vi "ModifyAcc.vi"(8 "error in (no error)":errorcluster, 11 "UserManagement in":refnum<class "UserManagement.lvclass">) -> (0 "error out":errorcluster, 3 "UserManagement out":refnum<class "UserManagement.lvclass">)   [LabVIEW 2019, in "UserManagement.lvlib" / "UserManagement.lvclass"]
uses:
  UserManagement.lvclass
  UserManagement.lvclass/UserManagement.ctl
panel:
  in  "Cancel":bool
  in  "OK":bool
  in  "RepeatPassWord":string
  in  "PassWord":string
  out "UesrName":string
  in  "Privileges":enum16{"Engineer", "Technical", "Operator"}(ring)
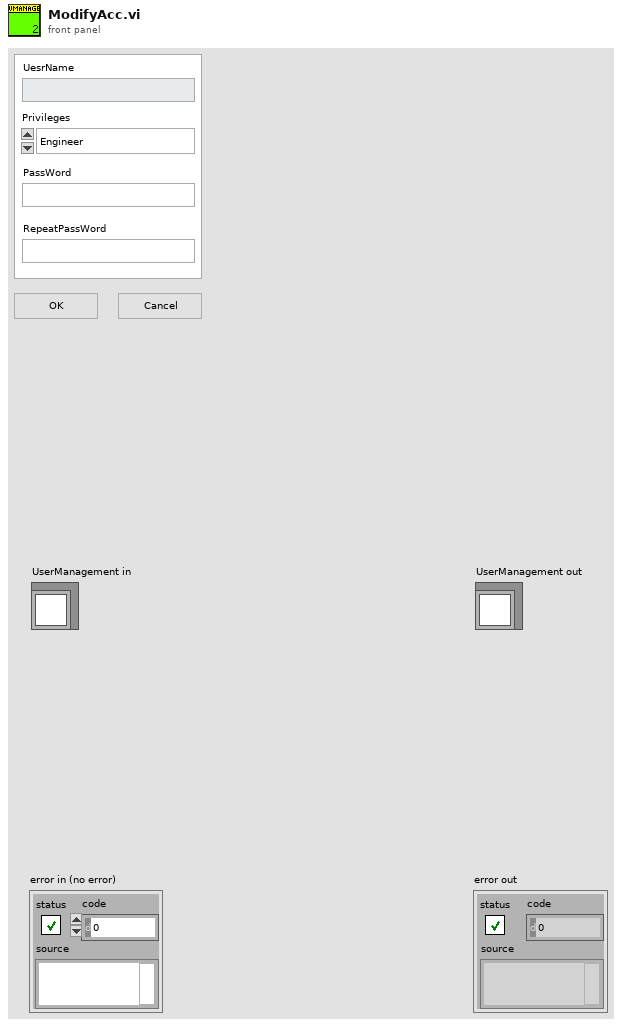
[diagram p1: front panel]
types:
  T1 = enum32{"Invalid", "Standard", "Closed", "Hidden", "Minimized", "Maximized"}
  T2 = enum32{"invalid app kind", "Development System", "Run Time System", "Student Edition", "Embedded LabVIEW", "Evaluation", "Custom"}
  T3 = cluster{"Core":cluster{"Current VI Reference":refnum<vi>, "Close Panel on Exit?":bool}, "Privileges":refnum<vi>, "Acc_Info_Str":string[][], "UserName":string, "Index":i32}
  T4 = cluster{"Current VI Reference":refnum<vi>, "Close Panel on Exit?":bool}
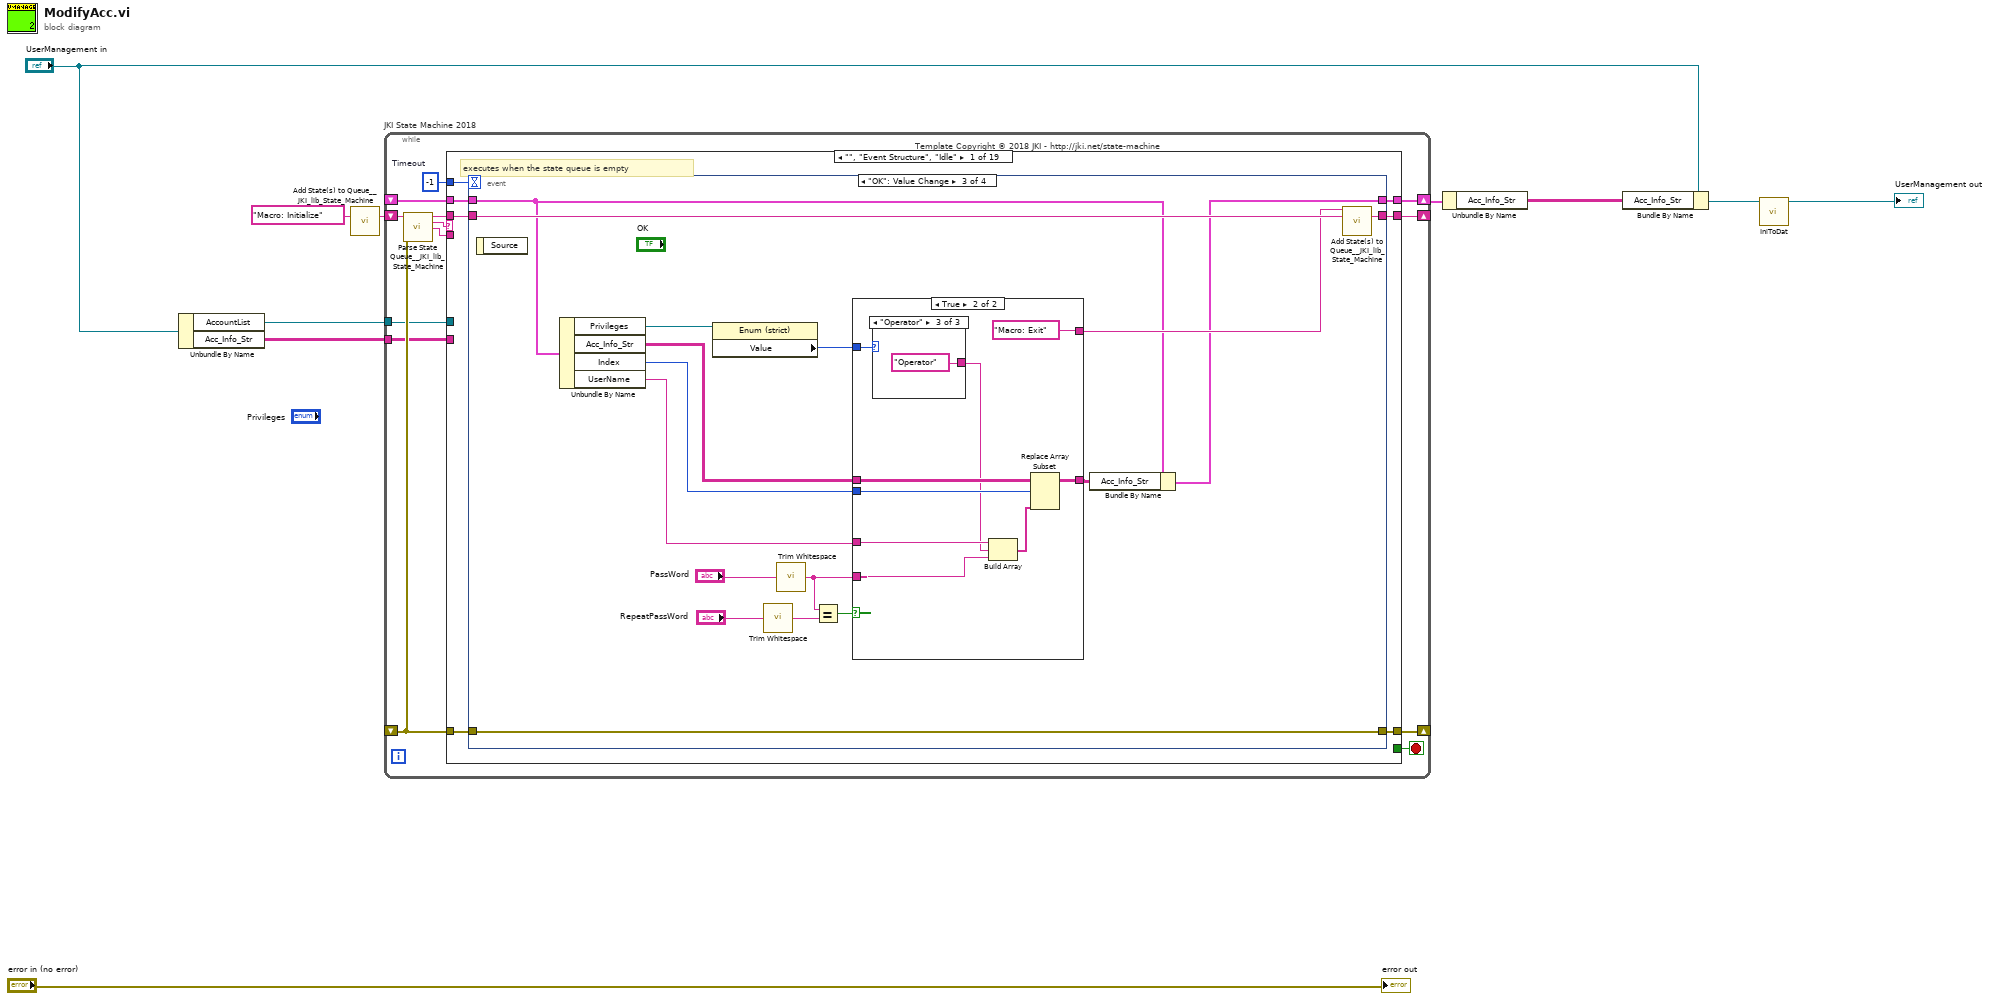
[diagram p0: block diagram]
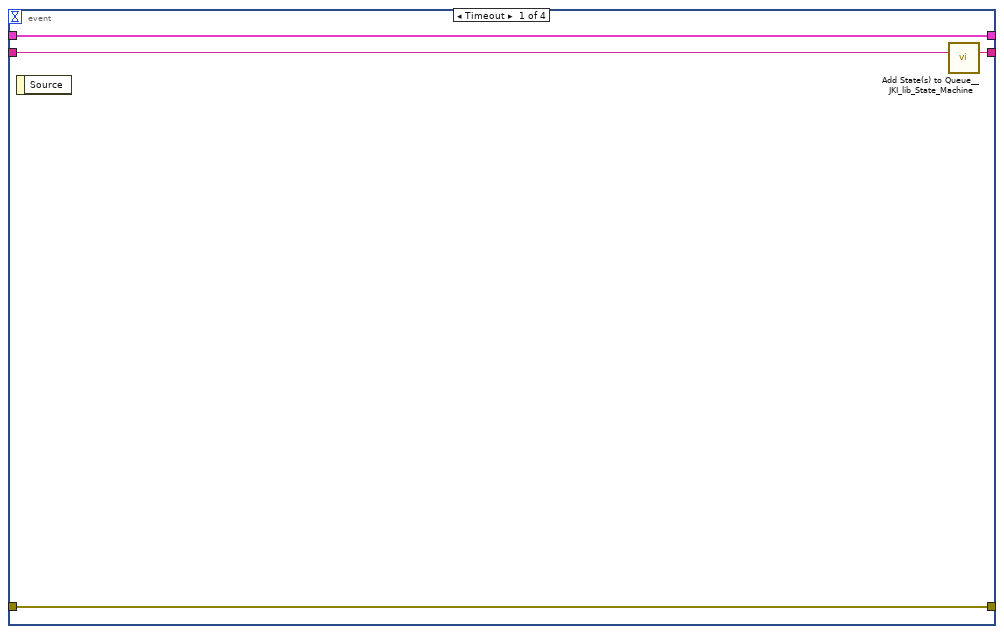
[diagram p2: hidden frame]
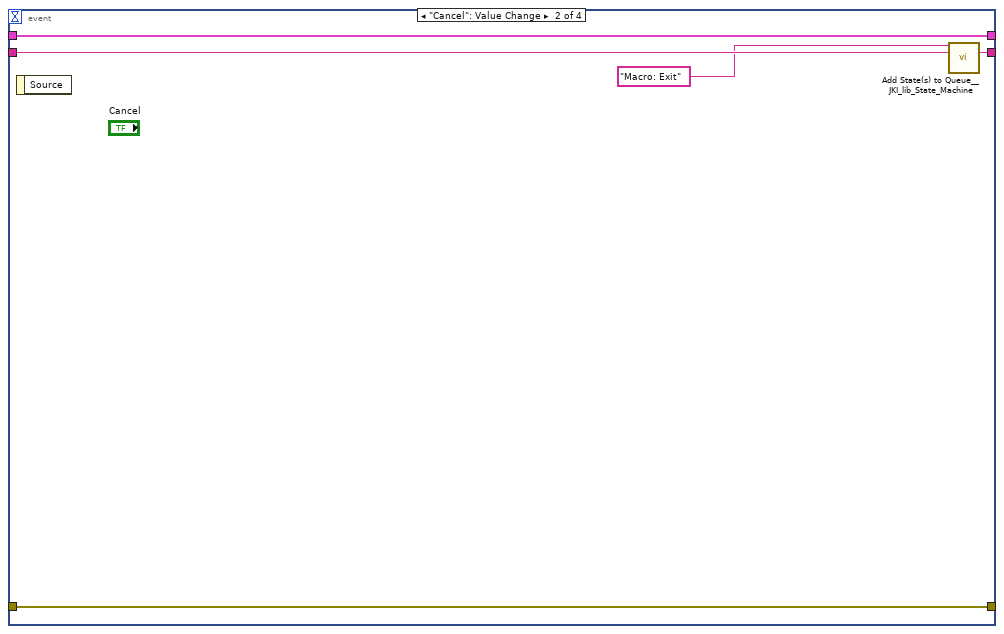
[diagram p3: hidden frame]
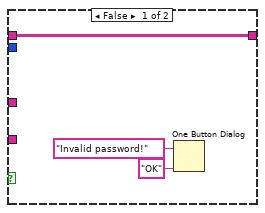
[diagram p4: hidden frame]
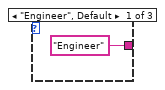
[diagram p5: hidden frame]
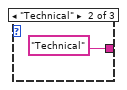
[diagram p6: hidden frame]
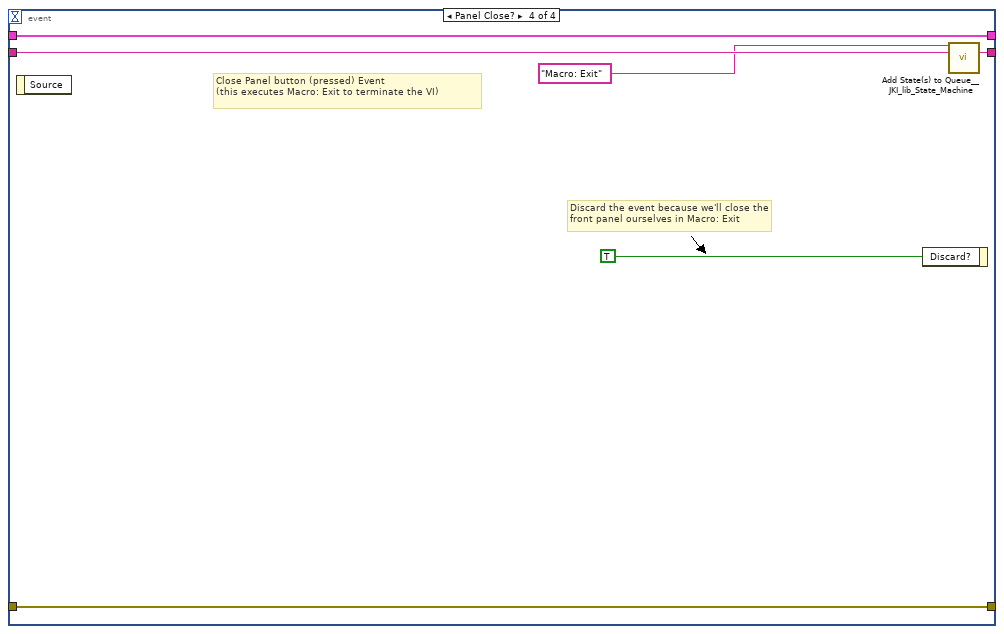
[diagram p7: hidden frame]
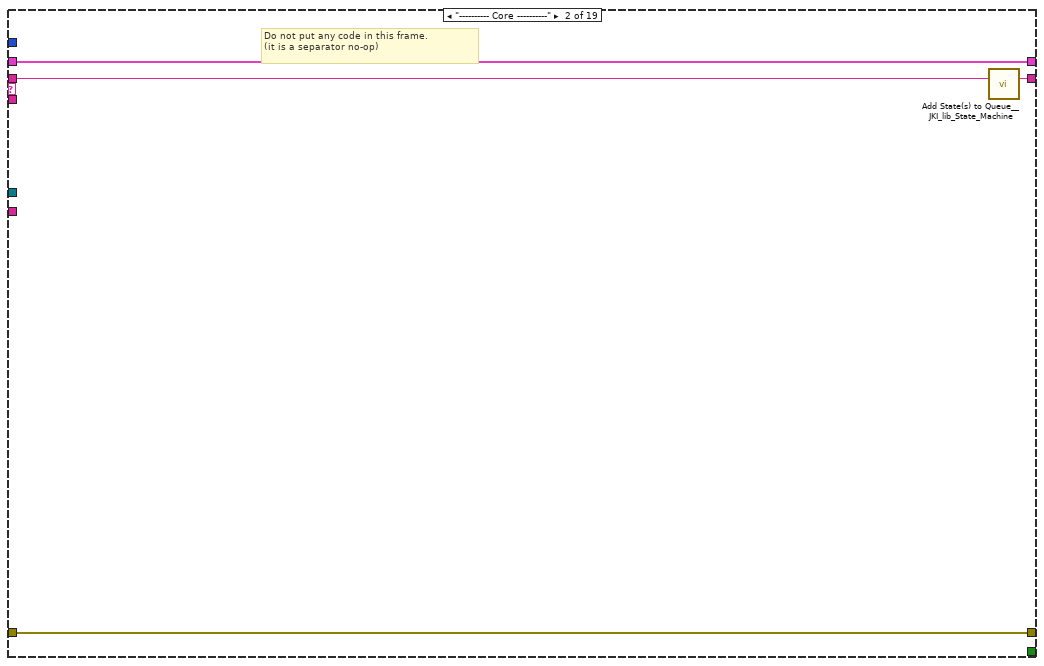
[diagram p8: hidden frame]
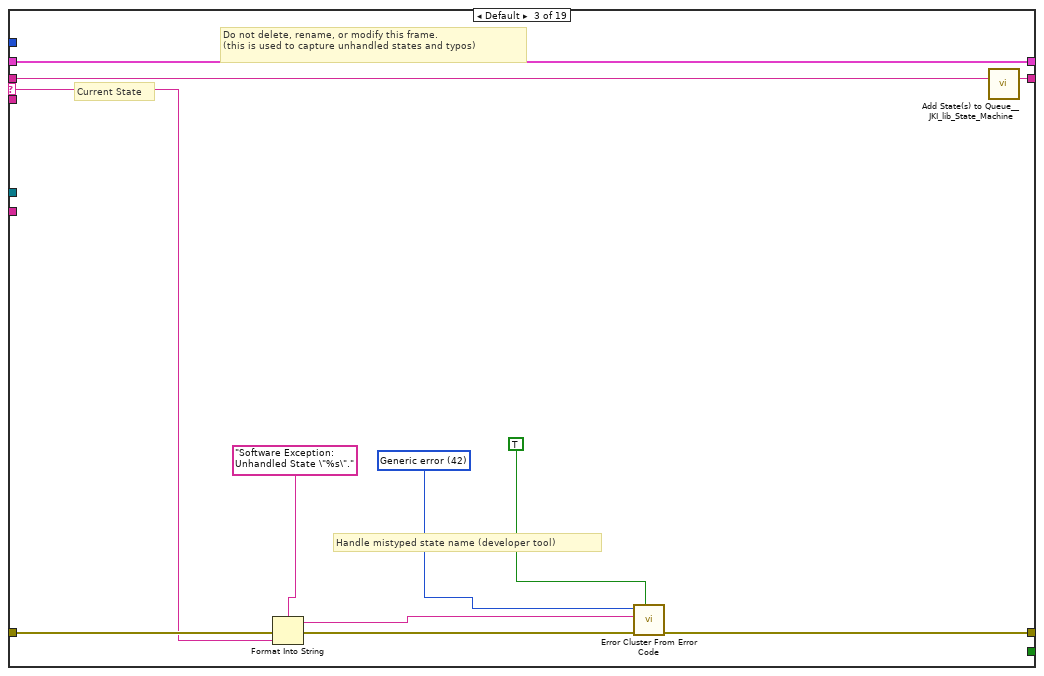
[diagram p9: hidden frame]
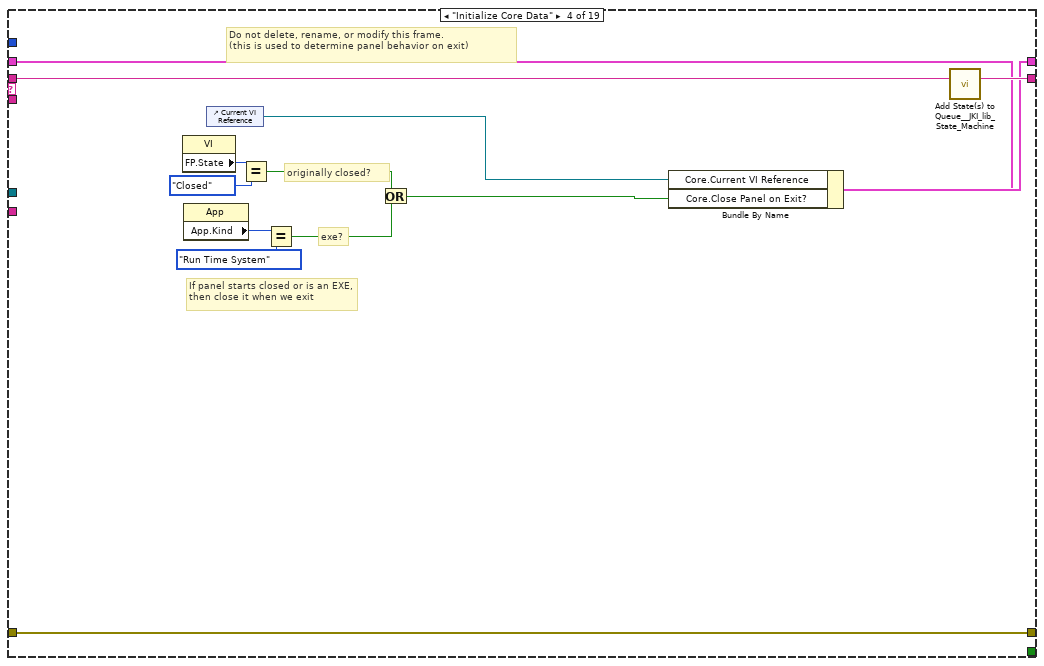
[diagram p10: hidden frame]
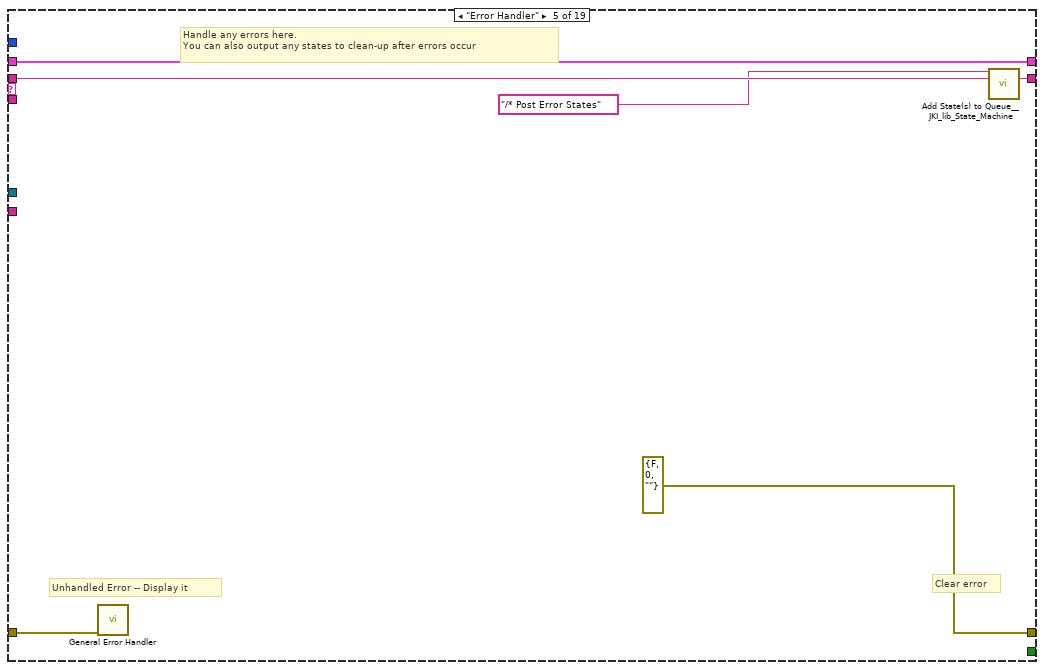
[diagram p11: hidden frame]
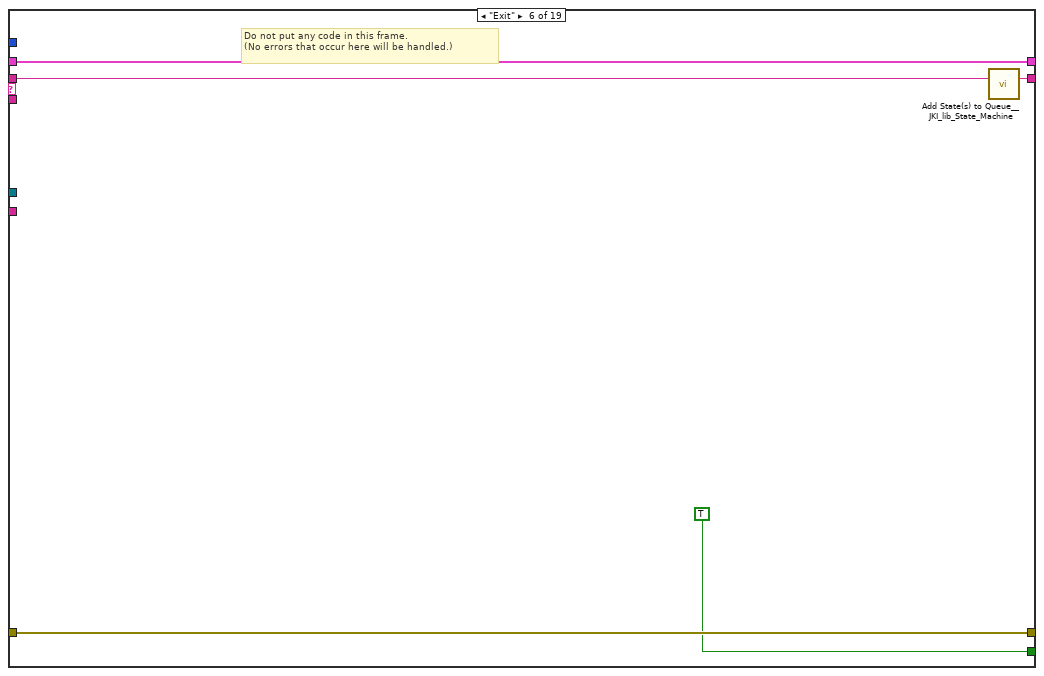
[diagram p12: hidden frame]
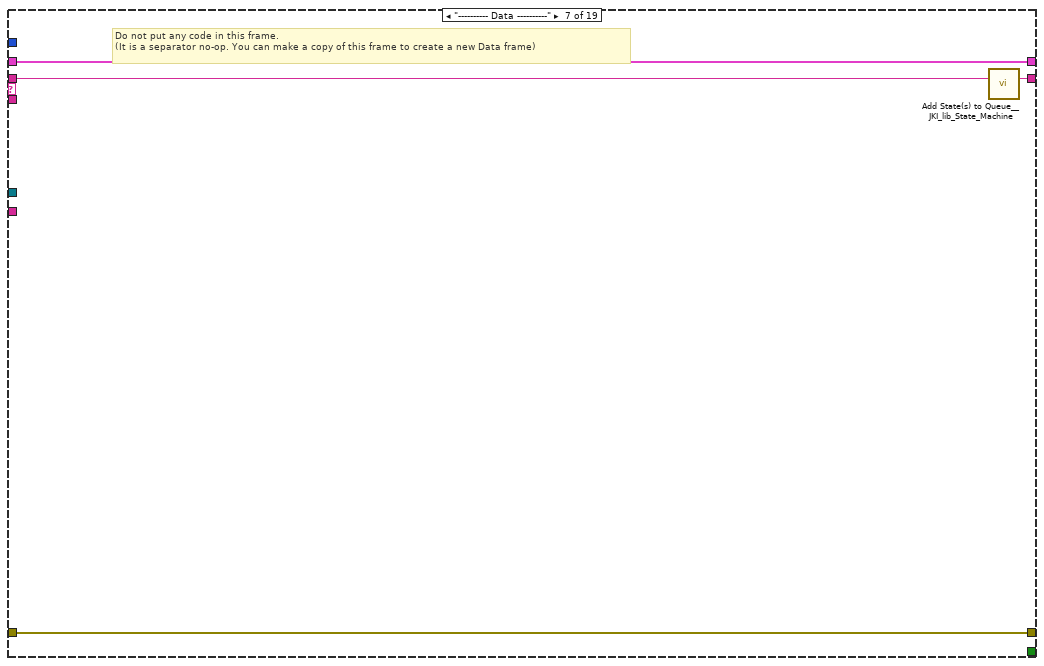
[diagram p13: hidden frame]
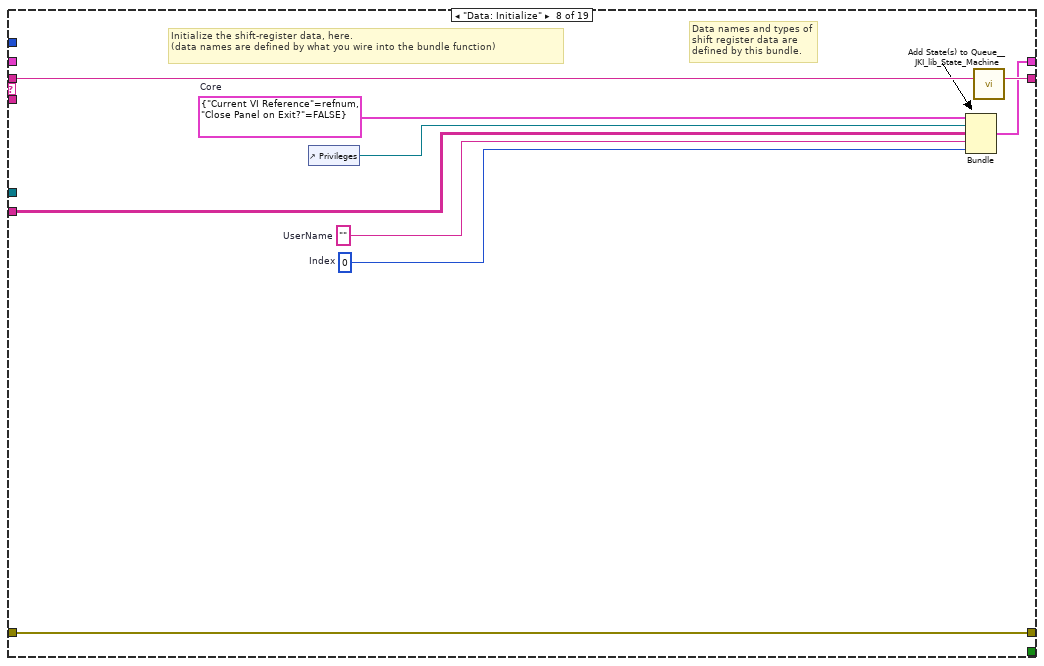
[diagram p14: hidden frame]
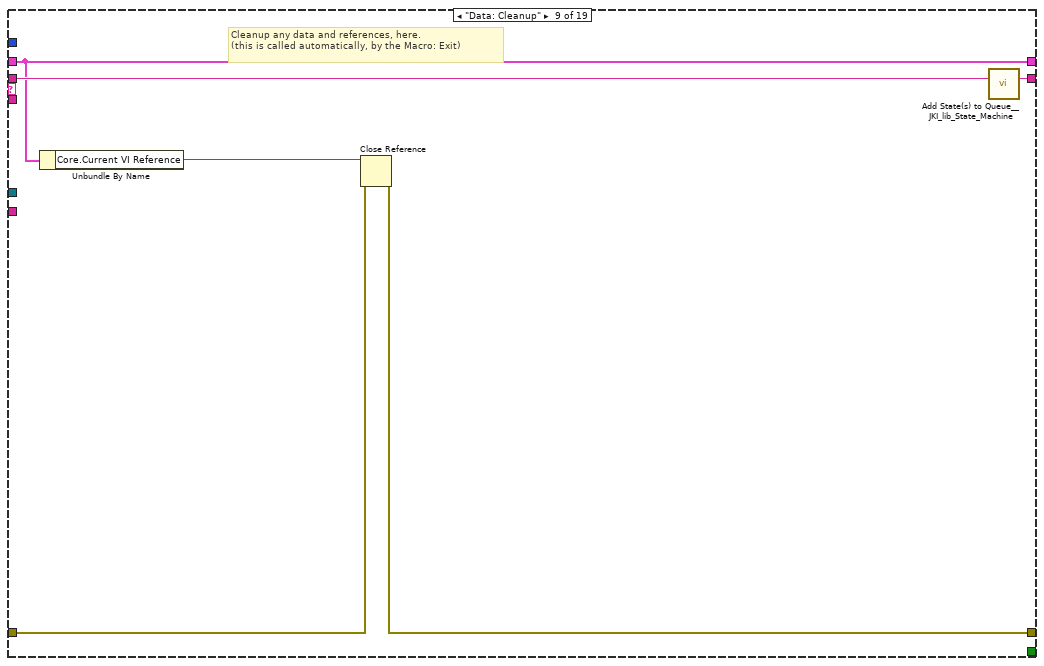
[diagram p15: hidden frame]
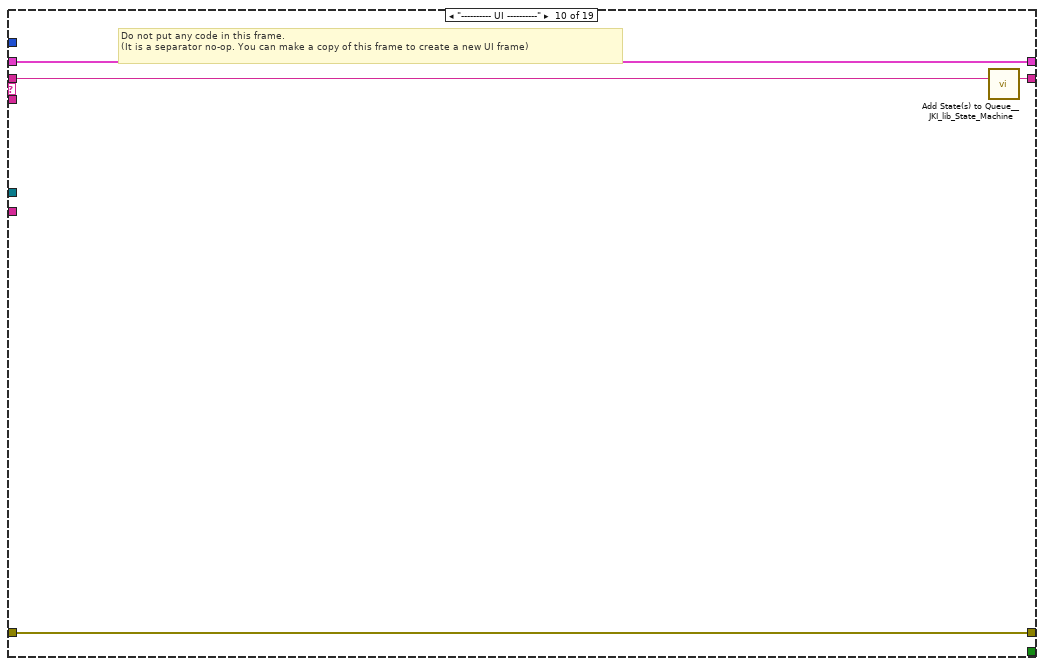
[diagram p16: hidden frame]
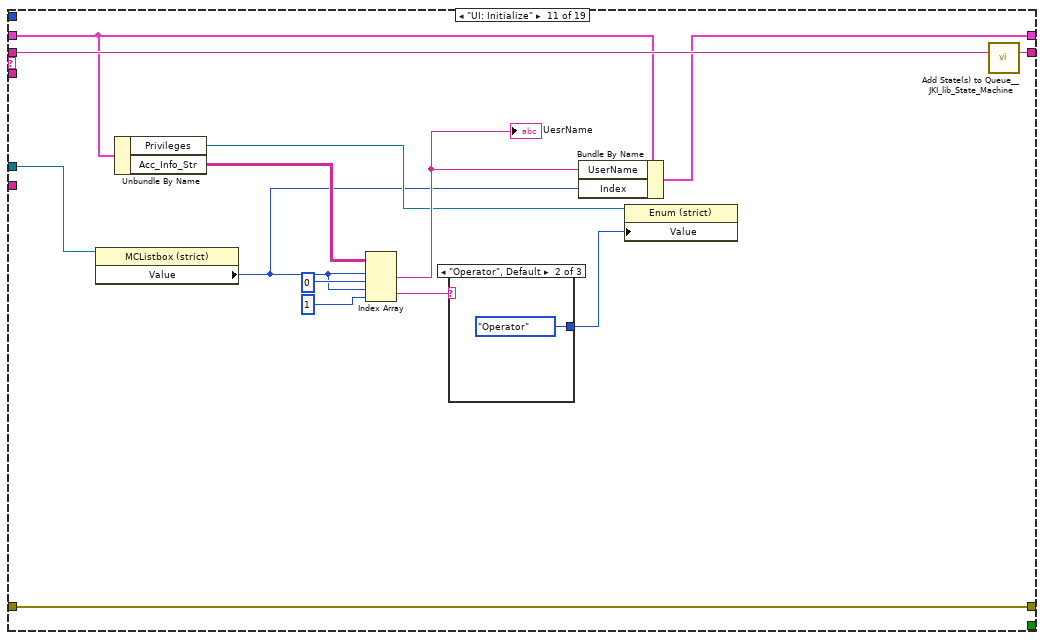
[diagram p17: hidden frame]
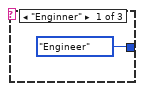
[diagram p18: hidden frame]
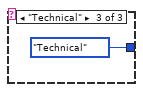
[diagram p19: hidden frame]
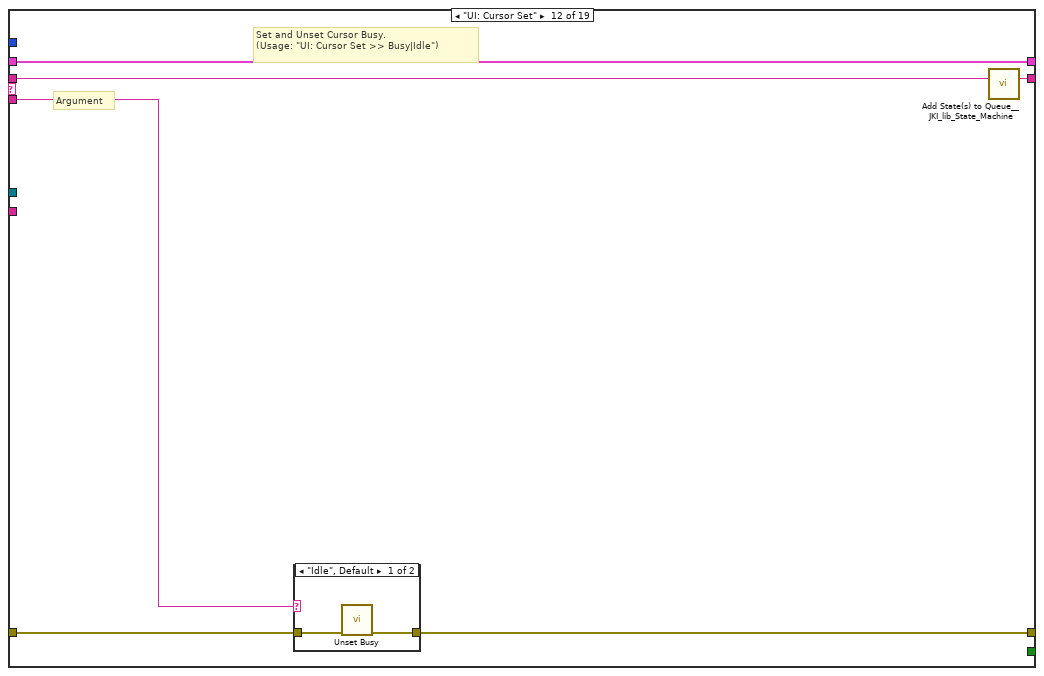
[diagram p20: hidden frame]
diagram:
  n1 = Unbundle By Name("UserManagement in") -> ("AccountList"=w7:refnum<vi>, "Acc_Info_Str"=w6:string[][])
  n2 = call <vilib>:"Add State(s) to Queue__JKI_lib_State_Machine.vi"("State(s) in (\"\")"="Macro: Initialize") -> ("States Out"=w9:string)  [unwired: 14 in]
  n3 = while "JKI State Machine 2018" {
    shift-right: [w16] -> w5
    shift-left: _ -> [w15]
    shift-right: [w19] -> _
    shift-left: _ -> [w13]
    shift-right: [w18] -> _
    shift-left: w9 -> [w20]
    tunnel: w7 -> [w12]
    tunnel: w6 -> [w11]
    stop <- w17 stop-if-true
    w14 = -1  # Timeout
    # "Template Copyright © 2018 JKI - http://jki.net/state-machine"
    n4 = call <vilib>:"Parse State Queue__JKI_lib_State_Machine.vi"("State Queue"=w20, "Error In (no error)"=w13) -> ("Remaining States"=w22:string, "Current State"=w23:string, "Arguments"=w21:string)  [unwired: 11 in]
    n5 = case shown="\"\", \"Event Structure\", \"Idle\"" w23 {
      selector: w23 -> [_ _ w82 _ _ _ _ _ _ _ _ _ _ _ _ _ _ _ _]
      tunnel: w22 -> [w30 w81 w86 w105 w111 w116 w120 w129 w135 w139 w153 w162 w173 w242 w247 w257 w261 w265 w269]
      tunnel: w21 -> [_ _ _ _ _ _ _ _ _ _ _ w157 w167 _ _ _ _ _ _]
      tunnel: w15 -> [w28 w78 w84 w98 w108 w114 w117 _ w130 w136 w144 w160 w169 w239 w244 w254 w258 w262 w266]
      tunnel: [w27 w79 w88 w102 errorcluster {"status"=FALSE, "code"=0, "source"=""} ("error out") w113 w118 w126 w131 w137 w151 w158 w170 w240 w245 w255 w259 w263 w267] -> w19
      tunnel: w13 -> [w26 w79 w87 w102 w107 w113 w118 w126 w132 w137 w151 w159 w171 w240 w245 w255 w259 w263 w267]
      tunnel: [w29 w80 w85 w104 w110 w115 w119 w128 w134 w138 w152 w161 w172 w241 w246 w256 w260 w264 w268] -> w18
      tunnel: [_ _ _ _ _ TRUE _ _ _ _ _ _ _ _ _ _ _ _ _] -> w17
      tunnel: [w25 w78 w84 w103 w108 w114 w117 w127 w130 w136 w141 w160 w169 w239 w244 w254 w258 w262 w266] -> w16
      tunnel: w14 -> [w24 _ _ _ _ _ _ _ _ _ _ _ _ _ _ _ _ _ _]
      tunnel: w12 -> [_ _ _ _ _ _ _ _ _ _ w142 _ _ _ _ _ _ _ _]
      tunnel: w11 -> [_ _ _ _ _ _ _ w123 _ _ _ _ _ _ _ _ _ _ _]
      frame "", "Event Structure", "Idle" {
        # "executes when the state queue is empty"
        n6 = event shown="[2] \"OK\": Value Change" {
          selector: _ -> [_ _ _ _]
          dyn-events: _ -> [_ _ _ _]
          timeout: w24 -> [_ _ _ _]
          tunnel: w30 -> [w34 w39 w56 w77]
          tunnel: [w33 w38 w55 w76] -> w29
          tunnel: w28 -> [w31 w36 w41 w74]
          tunnel: [w32 w37 w54 w75] -> w27
          tunnel: w26 -> [w32 w37 w54 w75]
          tunnel: [w31 w36 w40 w74] -> w25
          event Timeout {
            n7 = event-data() -> ()  [unwired: 1 in, 1 out]
            n8 = call <vilib>:"Add State(s) to Queue__JKI_lib_State_Machine.vi"("State(s) in (\"\")"=w34) -> ("States Out"=w33:string)  [unwired: 14 in]
          }
          event "Cancel": Value Change {
            n9 = event-data() -> ()  [unwired: 1 in, 1 out]
            n10 = call <vilib>:"Add State(s) to Queue__JKI_lib_State_Machine.vi"("State(s) in Front (\"\")"="Macro: Exit", "State(s) in (\"\")"=w39) -> ("States Out"=w38:string)  [unwired: 13 in]
          }
          event "OK": Value Change {
            n11 = event-data() -> ()  [unwired: 1 in, 1 out]
            n12 = Unbundle By Name(w41) -> ("Privileges"=w46:refnum<vi>, "Acc_Info_Str"=w45:string[][], "Index"=w44:i32, "UserName"=w43:string)
            n13 = property class="Enum (strict)"(reference=w46) -> ("Value"=w50:enum16{"Engineer", "Technical", "Operator"})  [unwired: 1 in, 2 out]
            n14 = call <vilib>:"Trim Whitespace.vi"("string"="RepeatPassWord") -> ("trimmed string"=w53:string)  [unwired: 1 in]
            n15 = call <vilib>:"Trim Whitespace.vi"("string"="PassWord") -> ("trimmed string"=w51:string)  [unwired: 1 in]
            n16 = Equal?(x=w51, y=w53) -> (x = y?=w52:bool)
            n17 = case shown="True" w52 {
              tunnel: w45 -> [w59 w68]
              tunnel: w44 -> [_ w67]
              tunnel: w51 -> [_ w62]
              tunnel: w43 -> [_ w64]
              tunnel: w50 -> [_ w66]
              tunnel: [w59 w65] -> w49
              tunnel: [_ "Macro: Exit"] -> w42
              frame False {
                n18 = One Button Dialog(message="Invalid password!" ("消息"), button name ("OK")="OK" ("按钮名称（“确定”）")) -> ()  [unwired: 1 out]
              }
              frame True {
                n19 = case shown="\"Operator\"" w66 {
                  tunnel: ["Engineer" "Technical" "Operator"] -> w63
                  frame "Engineer", Default {
                  }
                  frame "Technical" {
                  }
                  frame "Operator" {
                  }
                }
                n20 = Build Array(w64, w63, w62) -> (w61:string[])
                n21 = Replace Array Subset(array=w68, new element=w61, index (row)=w67) -> (w65:string[][])  [unwired: 1 in]
              }
            }
            n22 = Bundle By Name(cluster=w41, "Acc_Info_Str"=w49) -> (w40:T3)
            n23 = call <vilib>:"Add State(s) to Queue__JKI_lib_State_Machine.vi"("State(s) in Front (\"\")"=w42, "State(s) in (\"\")"=w56) -> ("States Out"=w55:string)  [unwired: 13 in]
          }
          event Panel Close? {
            # "Discard the event because we'll close the front panel ourselves in Macro: Exit"
            # "Close Panel button (pressed) Event\n(this executes Macro: Exit to terminate the VI)"
            n24 = event-data() -> ()  [unwired: 1 in, 1 out]
            n25 = event-data("Discard?"=TRUE) -> ()  [unwired: 1 in, 1 out]
            n26 = call <vilib>:"Add State(s) to Queue__JKI_lib_State_Machine.vi"("State(s) in Front (\"\")"="Macro: Exit", "State(s) in (\"\")"=w77) -> ("States Out"=w76:string)  [unwired: 13 in]
          }
        }
      }
      frame "---------- Core ----------" {
        # "Do not put any code in this frame.\n(it is a separator no-op)"
        n27 = call <vilib>:"Add State(s) to Queue__JKI_lib_State_Machine.vi"("State(s) in (\"\")"=w81) -> ("States Out"=w80:string)  [unwired: 14 in]
      }
      frame Default {
        w91 = 42 items=["No error", "Argument error", "Memory is full", "Out of zone", "End of file", "File already open", "Generic file I/O error", "File not found", "File permission error", "Disk is full", "Duplicate path", "Too many files open", "System feature not enabled", "Resource file not found", "Cannot add resource", "Resource not found", "Image not found", "Image memory error", "Pen does not exist", "Config type invalid", "Config token not found", "Config parse error", "Config memory error", "Bad external code format", "Bad external code offset", "External code not present", "Null window", "Destroy window error", "Null menu", "Print aborted", "Bad print record", "Print driver error", "Windows error during printing", "Memory error during printing", "Print dialog error", "Generic print error", "Invalid device refnum", "Device not found", "Device parameter error", "Device unit error", "Cannot open device", "Device call aborted", "Generic error", "Cancelled by user", "Object ID too low", "Object ID too high", "Object not in heap", "Unknown heap", "Unknown object (invalid DefProc)", "Unknown object (DefProc not in table)", "Message out of range", "Invalid (null) method", "Unknown message", "Manager call not supported", "Bad address", "Network operation in progress", "Network operation timed out", "Connection is busy", "Network attribute not supported", "Network error", "Address in use", "System out of memory", "Connection aborted", "Connection refused", "Not connected", "Already connected", "Connection closed", "Initialization error (interapplication manager)", "Bad occurrence", "Wait on unbound occurrence handler", "Occurrence queue overflow", "Datalog type conflict", "Unused", "Unrecognized type (interapplication manager)", "Memory corrupt", "Failed to make temporary DLL", "Old CIN version", "Drag socket not found", "Failed to load drop-object", "Failed to register OLE object", "Failed to release OLE object", "Format specifier type mismatch", "Unknown format specifier", "Too few format specifiers", "Too many format specifiers", "Scan failed", "Newer CIN version", "Error converting to variant", "Runtime menu error", "Password tampered", "Variant attribute not found", "Incompatible variant data type", "Event data is not available", "Event Store is not present", "Occurrence is not found", "Event Queue is not created", "Event info is not available", "Refnum passed is NULL", "Error retrieving Class GUID", "Error retrieving CoClass GUID", "Error retrieving TypeLib GUID.", "Bad built application magic bytes.", "Specific driver is different from the specific driver associated with the Logical Name.", "There is no session opened to the class driver.", "Max Error", "MAX - Error with config objects", "MAX - Error loading configuration", "MAX - Group not supported"]
        # "Current State"
        # "Do not delete, rename, or modify this frame.\n(this is used to capture unhandled states and typos)"
        # "Handle mistyped state name (developer tool)"
        n28 = Format Into String(format string="Software Exception: Unhandled State \"%s\"." ("message"), error in=w87, w82) -> (resulting string=w90:string, error out=w89:errorcluster)  [unwired: 1 in]
        n29 = call <vilib>:"Error Cluster From Error Code.vi"("show call chain? (False)"=TRUE, "error in (no error)"=w89, "error message (\"\")"=w90, "error code (0)"=w91) -> ("error out"=w88:errorcluster)  [unwired: 5 in]
        n30 = call <vilib>:"Add State(s) to Queue__JKI_lib_State_Machine.vi"("State(s) in (\"\")"=w86) -> ("States Out"=w85:string)  [unwired: 14 in]
      }
      frame "Initialize Core Data" {
        # "Do not delete, rename, or modify this frame.\n(this is used to determine panel behavior on exit)"
        # "originally closed?"
        # "exe?"
        # "If panel starts closed or is an EXE, then close it when we exit"
        n31 = property class="VI"() -> ("FP.State"=w95:T1)  [unwired: 2 in, 2 out]
        n32 = property class="App"() -> ("App.Kind"=w101:T2)  [unwired: 2 in, 2 out]
        n33 = control-ref of="Current VI Reference"() -> (w96:refnum<vi>)
        n34 = Equal?(x=w95, y=T1."Closed" ("Front Panel Window:State")) -> (x = y?=w93:bool)
        n35 = Equal?(x=w101, y=T2."Run Time System" ("Application:Kind")) -> (x = y?=w99:bool)
        n36 = Or(x=w93, y=w99) -> (x .or. y?=w97:bool)
        n37 = Bundle By Name(cluster=w98, "Core.Current VI Reference"=w96, "Core.Close Panel on Exit?"=w97) -> (w103:T3)
        n38 = call <vilib>:"Add State(s) to Queue__JKI_lib_State_Machine.vi"("State(s) in (\"\")"=w105) -> ("States Out"=w104:string)  [unwired: 14 in]
      }
      frame "Error Handler" {
        # "Unhandled Error -- Display it"
        # "Handle any errors here.\nYou can also output any states to clean-up after errors occur"
        # "Clear error"
        n39 = call <vilib>:"General Error Handler.vi"("error in (no error)"=w107) -> ()  [unwired: 10 in, 5 out]
        n40 = call <vilib>:"Add State(s) to Queue__JKI_lib_State_Machine.vi"("State(s) in Front (\"\")"="/* Post Error States", "State(s) in (\"\")"=w111) -> ("States Out"=w110:string)  [unwired: 13 in]
      }
      frame "Exit" {
        # "Do not put any code in this frame.\n(No errors that occur here will be handled.)"
        n41 = call <vilib>:"Add State(s) to Queue__JKI_lib_State_Machine.vi"("State(s) in (\"\")"=w116) -> ("States Out"=w115:string)  [unwired: 14 in]
      }
      frame "---------- Data ----------" {
        # "Do not put any code in this frame.\n(It is a separator no-op. You can make a copy of this frame to create a new Data frame)"
        n42 = call <vilib>:"Add State(s) to Queue__JKI_lib_State_Machine.vi"("State(s) in (\"\")"=w120) -> ("States Out"=w119:string)  [unwired: 14 in]
      }
      frame "Data: Initialize" {
        w121 = 0  # Index
        w122 = ""  # UserName
        w125 = T4 {"Current VI Reference"=refnum, "Close Panel on Exit?"=FALSE}  # Core
        # "Data names and types of shift register data are defined by this bundle."
        # "Initialize the shift-register data, here.\n(data names are defined by what you wire into the bundle function)"
        n43 = control-ref of="Privileges"() -> (w124:refnum<vi>)
        n44 = Bundle("Core"=w125, "Privileges"=w124, "Acc_Info_Str"=w123, "UserName"=w122, "Index"=w121) -> (w127:T3)  [unwired: 1 in]
        n45 = call <vilib>:"Add State(s) to Queue__JKI_lib_State_Machine.vi"("State(s) in (\"\")"=w129) -> ("States Out"=w128:string)  [unwired: 14 in]
      }
      frame "Data: Cleanup" {
        # "Cleanup any data and references, here.\n(this is called automatically, by the Macro: Exit)"
        n46 = Unbundle By Name(w130) -> ("Core.Current VI Reference"=w133:refnum<vi>)
        n47 = Close Reference(reference=w133, error in (no error)=w132) -> (error out=w131:errorcluster)
        n48 = call <vilib>:"Add State(s) to Queue__JKI_lib_State_Machine.vi"("State(s) in (\"\")"=w135) -> ("States Out"=w134:string)  [unwired: 14 in]
      }
      frame "---------- UI ----------" {
        # "Do not put any code in this frame.\n(It is a separator no-op. You can make a copy of this frame to create a new UI frame)"
        n49 = call <vilib>:"Add State(s) to Queue__JKI_lib_State_Machine.vi"("State(s) in (\"\")"=w139) -> ("States Out"=w138:string)  [unwired: 14 in]
      }
      frame "UI: Initialize" {
        n50 = property class="MCListbox (strict)"(reference=w142) -> ("Value"=w140:i32)  [unwired: 1 in, 2 out]
        n51 = Unbundle By Name(w144) -> ("Privileges"=w145:refnum<vi>, "Acc_Info_Str"=w143:string[][])
        n52 = Index Array(array=w143, index (row) #1=w140, index (col) #1=0 ("禁用的索引 (列)"), index (row) #2=w140, index (col) #2=1 ("禁用的索引 (列)")) -> (element #1=w146:string, element #2=w148:string)
        "UesrName" <- w146
        n53 = case shown="\"Operator\", Default" w148 {
          tunnel: [enum16{"Engineer", "Technical", "Operator"}."Engineer" ("Value") enum16{"Engineer", "Technical", "Operator"}."Operator" ("Value") enum16{"Engineer", "Technical", "Operator"}."Technical" ("Value")] -> w147
          frame "Enginner" {
          }
          frame "Operator", Default {
          }
          frame "Technical" {
          }
        }
        n54 = Bundle By Name(cluster=w144, "UserName"=w146, "Index"=w140) -> (w141:T3)
        n55 = property class="Enum (strict)"(reference=w145, "Value"=w147) -> ()  [unwired: 1 in, 2 out]
        n56 = call <vilib>:"Add State(s) to Queue__JKI_lib_State_Machine.vi"("State(s) in (\"\")"=w153) -> ("States Out"=w152:string)  [unwired: 14 in]
      }
      frame "UI: Cursor Set" {
        # "Argument"
        # "Set and Unset Cursor Busy.\n(Usage: \"UI: Cursor Set >> Busy|Idle\")"
        n57 = case shown="\"Idle\", Default" w157 {
          tunnel: w159 -> [w164 w166]
          tunnel: [w163 w165] -> w158
          frame "Idle", Default {
            n58 = call <vilib>:"Unset Busy.vi"("error in (no error)"=w164) -> ("error out"=w163:errorcluster)  [unwired: 10 in]
          }
          frame "Busy" {
            n59 = call <vilib>:"Set Busy.vi"("error in (no error)"=w166) -> ("error out"=w165:errorcluster)  [unwired: 9 in, 1 out]
          }
        }
        n60 = call <vilib>:"Add State(s) to Queue__JKI_lib_State_Machine.vi"("State(s) in (\"\")"=w162) -> ("States Out"=w161:string)  [unwired: 14 in]
      }
      frame "UI: Front Panel State" {
        # "Argument"
        # "Set Front Panel Open or Closed\n(Usage: \"UI: Front Panel State >> Open|Close\")"
        n61 = Unbundle By Name(w169) -> ("Core.Current VI Reference"=w168:refnum<vi>)
        n62 = case shown="\"Minimize\", \"Minimized\"" w167 {
          tunnel: w171 -> [w179 w194 w205 w218 w231]
          tunnel: [w181 w195 w207 w220 w233] -> w170
          tunnel: w168 -> [w180 w192 w206 w219 w232]
          frame "Open", "Standard", Default {
            w174 = T1."Standard" ("State")
            n63 = property class="VI"(reference=w180, error in=w179) -> (reference out=w177:refnum<vi>, error out=w178:errorcluster, "FP.State"=w176:T1)
            n64 = Not Equal?(x=w176, y=w174) -> (x != y?=w175:bool)
            n65 = case shown="True" w175 {
              tunnel: [w185 w187] -> w181
              tunnel: w178 -> [w184 w187]
              tunnel: w177 -> [w183 _]
              tunnel: w174 -> [w182 _]
              frame True {
                n66 = invoke class="VI" method="FP.Open"(reference=w183, error in=w184, "Activate"=TRUE, "State"=w182) -> (error out=w185:errorcluster)  [unwired: 1 in, 4 out]
              }
              frame False {
              }
            }
          }
          frame "Close", "Closed" {
            n67 = property class="VI"(reference=w192, error in=w194) -> (reference out=w191:refnum<vi>, error out=w193:errorcluster, "FP.State"=w189:T1)
            n68 = Not Equal?(x=w189, y=T1."Closed" ("Front Panel Window:State")) -> (x != y?=w188:bool)
            n69 = case shown="True" w188 {
              tunnel: [w196 w199] -> w195
              tunnel: w193 -> [w196 w198]
              tunnel: w191 -> [_ w197]
              frame False {
              }
              frame True {
                n70 = invoke class="VI" method="FP.Close"(reference=w197, error in=w198) -> (error out=w199:errorcluster)  [unwired: 1 in, 2 out]
              }
            }
          }
          frame "Hidden", "Hide" {
            w200 = T1."Hidden" ("State")
            n71 = property class="VI"(reference=w206, error in=w205) -> (reference out=w203:refnum<vi>, error out=w204:errorcluster, "FP.State"=w202:T1)
            n72 = Not Equal?(x=w202, y=w200) -> (x != y?=w201:bool)
            n73 = case shown="True" w201 {
              tunnel: [w211 w212] -> w207
              tunnel: w204 -> [w210 w212]
              tunnel: w203 -> [w209 _]
              tunnel: w200 -> [w208 _]
              frame True {
                n74 = invoke class="VI" method="FP.Open"(reference=w209, error in=w210, "State"=w208) -> (error out=w211:errorcluster)  [unwired: 2 in, 4 out]
              }
              frame False {
              }
            }
          }
          frame "Minimize", "Minimized" {
            w213 = T1."Minimized" ("State")
            n75 = property class="VI"(reference=w219, error in=w218) -> (reference out=w216:refnum<vi>, error out=w217:errorcluster, "FP.State"=w215:T1)
            n76 = Not Equal?(x=w215, y=w213) -> (x != y?=w214:bool)
            n77 = case shown="True" w214 {
              tunnel: [w224 w225] -> w220
              tunnel: w217 -> [w223 w225]
              tunnel: w216 -> [w222 _]
              tunnel: w213 -> [w221 _]
              frame True {
                n78 = invoke class="VI" method="FP.Open"(reference=w222, error in=w223, "State"=w221) -> (error out=w224:errorcluster)  [unwired: 2 in, 4 out]
              }
              frame False {
              }
            }
          }
          frame "Maximize", "Maximized" {
            w226 = T1."Maximized" ("State")
            n79 = property class="VI"(reference=w232, error in=w231) -> (reference out=w229:refnum<vi>, error out=w230:errorcluster, "FP.State"=w228:T1)
            n80 = Not Equal?(x=w228, y=w226) -> (x != y?=w227:bool)
            n81 = case shown="True" w227 {
              tunnel: [w237 w238] -> w233
              tunnel: w230 -> [w236 w238]
              tunnel: w229 -> [w235 _]
              tunnel: w226 -> [w234 _]
              frame True {
                n82 = invoke class="VI" method="FP.Open"(reference=w235, error in=w236, "State"=w234) -> (error out=w237:errorcluster)  [unwired: 2 in, 4 out]
              }
              frame False {
              }
            }
          }
        }
        n83 = call <vilib>:"Add State(s) to Queue__JKI_lib_State_Machine.vi"("State(s) in (\"\")"=w173) -> ("States Out"=w172:string)  [unwired: 14 in]
      }
      frame "---------- Macro ----------" {
        # "Do not put any code in this frame.\n(It is a separator no-op. You can make a copy of this frame to create a new Macro frame)"
        n84 = call <vilib>:"Add State(s) to Queue__JKI_lib_State_Machine.vi"("State(s) in (\"\")"=w242) -> ("States Out"=w241:string)  [unwired: 14 in]
      }
      frame "Macro: Initialize" {
        w243 = "Data: Initialize\nInitialize Core Data\nUI: Initialize\nUI: Front Panel State >> Open"  # Data: Initialize Initialize Core Data UI: Initialize UI: Front Panel State >> Open
        # "Initialization Macro\n(This is called once, when the VI starts)"
        n85 = call <vilib>:"Add State(s) to Queue__JKI_lib_State_Machine.vi"("State(s) in Front (\"\")"=w243, "State(s) in (\"\")"=w247) -> ("States Out"=w246:string)  [unwired: 13 in]
      }
      frame "Macro: Exit" {
        # "Exit Macro\n(This is called once, when the VI exits)"
        n86 = Unbundle By Name(w254) -> ("Core.Close Panel on Exit?"=w253:bool)
        n87 = Select(t="UI: Front Panel State >> Close", s=w253, f="") -> (s? t:f=w250:string)
        n88 = call <vilib>:"Add State(s) to Queue__JKI_lib_State_Machine.vi"("State(s) in (\"\")"=w250, "State(s) at Back (\"\")"="Data: Cleanup\nExit") -> ("States Out"=w248:string)  [unwired: 13 in]
        n89 = call <vilib>:"Add State(s) to Queue__JKI_lib_State_Machine.vi"("State(s) in Front (\"\")"=w248, "State(s) in (\"\")"=w257) -> ("States Out"=w256:string)  [unwired: 13 in]
      }
      frame "---------- New Category ----------" {
        # "Template Separator\n(You can make a copy of, or modify, this frame)"
        n90 = call <vilib>:"Add State(s) to Queue__JKI_lib_State_Machine.vi"("State(s) in (\"\")"=w261) -> ("States Out"=w260:string)  [unwired: 14 in]
      }
      frame "New Category: 1" {
        # "Your code here.\n(You can make a copy of, or modify, this frame)"
        n91 = call <vilib>:"Add State(s) to Queue__JKI_lib_State_Machine.vi"("State(s) in (\"\")"=w265) -> ("States Out"=w264:string)  [unwired: 14 in]
      }
      frame "New Category: 2" {
        # "Your code here.\n(You can make a copy of, or modify, this frame)"
        n92 = call <vilib>:"Add State(s) to Queue__JKI_lib_State_Machine.vi"("State(s) in (\"\")"=w269) -> ("States Out"=w268:string)  [unwired: 14 in]
      }
    }
  }
  n93 = Unbundle By Name(w5) -> ("Acc_Info_Str"=w3:string[][])
  n94 = Bundle By Name(cluster="UserManagement in", "Acc_Info_Str"=w3) -> (w2:refnum<class "UserManagement.lvclass">)
  n95 = call-dynamic "IniToDat.vi"("UserManagement in"=w2) -> ("UserManagement out"=→"UserManagement out":refnum<class "UserManagement.lvclass">)  [unwired: 9 in, 1 out]
  "error out" <- "error in (no error)"
